vi "Configure Slot.vi"(6 "Delay (sec)":dbl min=0.0 max=99999.999 format="%#.3f", 7 "Number of Poles (1)":enum16{"1", "2", "4"}(ring), 8 "error in":errorcluster, 9 "Card Type (None)":T1(ring), 10 "Slot # (1)":u32=1 min=1 max=2, 11 "VISA resource name":refnum<visa-resource-name>) -> (0 "error out":errorcluster, 3 "VISA resource name out":refnum<visa-resource-name>)   [LabVIEW 2018, in "Keithley 7001.lvlib"]
uses:
  <instrlib>/Keithley 7001/Keithley 7001.lvlib
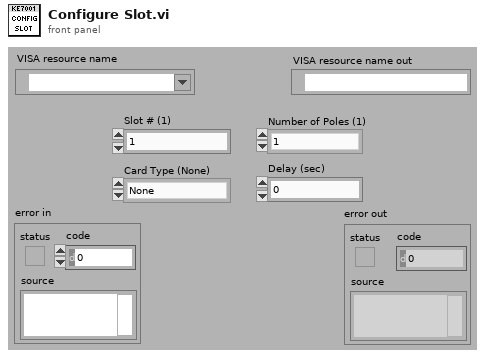
[diagram p1: front panel]
types:
  T1 = enum16{"None", "7052", "7053", "7054", "7056", "7057", "7058", "7059", "7061", "7062", "7063", "7064", "7065", "7066", "7067", "7152", "7153", "7154", "7156", "7158", "7164", "7166", "7168", "7169", "7402", "9990", "9991"}
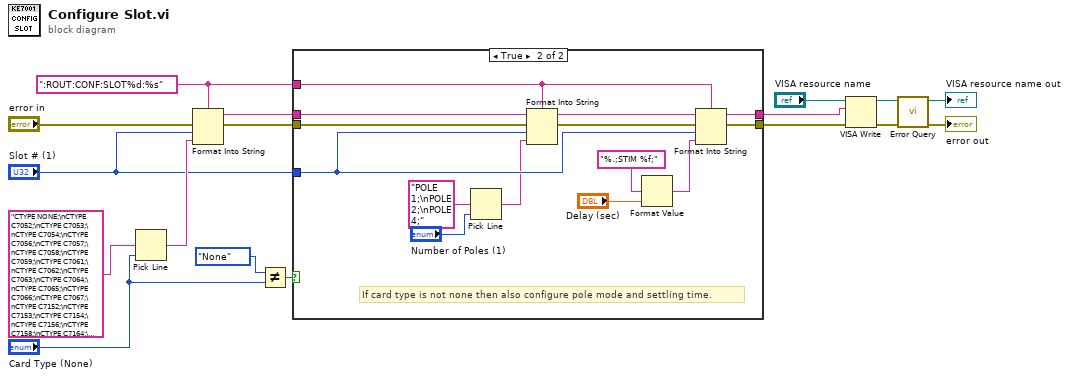
[diagram p0: block diagram]
diagram:
  w8 = ":ROUT:CONF:SLOT%d:%s" ("format string")
  n1 = Pick Line(multi-line string="CTYPE NONE;\nCTYPE C7052;\nCTYPE C7053;\nCTYPE C7054;\nCTYPE C7056;\nCTYPE C7057;\nCTYPE C7058;\nCTYPE C7059;\nCTYPE C7061;\nCTYPE C7062;\nCTYPE C7063;\nCTYPE C7064;\nCTYPE C7065;\nCTYPE C7066;\nCTYPE C7067;\nCTYPE C7152;\nCTYPE C7153;\nCTYPE C7154;\nCTYPE C7156;\nCTYPE C7158;\nCTYPE C7164;\nCTYPE C7166;\nCTYPE C7168;\nCTYPE C7169;\nCTYPE C7402;\nCTYPE C9990;\nCTYPE C9991;", line index="Card Type (None)") -> (output string=w12:string)  [unwired: 1 in]
  n2 = Format Into String(format string=w8, error in="error in", "Slot # (1)", w12) -> (resulting string=w10:string, error out=w9:errorcluster)  [unwired: 1 in]
  n3 = Not Equal?(x=T1."None", y="Card Type (None)") -> (x != y?=w7:bool)
  n4 = case shown="True" w7 {
    tunnel: w10 -> [w19 w30]
    tunnel: w9 -> [w18 w29]
    tunnel: w8 -> [_ w28]
    tunnel: "Slot # (1)" -> [_ w26]
    tunnel: [w19 w22] -> w2
    tunnel: [w18 w20] -> w1
    frame False {
      # "If the card type is None then don't configure pole mode\nor settling time."
    }
    frame True {
      # "If card type is not none then also configure pole mode and settling time."
      n5 = Pick Line(multi-line string="POLE 1;\nPOLE 2;\nPOLE 4;", line index="Number of Poles (1)") -> (output string=w24:string)  [unwired: 1 in]
      n6 = Format Into String(format string=w28, initial string=w30, error in=w29, w26, w24) -> (resulting string=w21:string, error out=w23:errorcluster)
      n7 = Format Value(format string="%.;STIM %f;", value (0)="Delay (sec)") -> (output string=w27:string)  [unwired: 1 in]
      n8 = Format Into String(format string=w28, initial string=w21, error in=w23, w26, w27) -> (resulting string=w22:string, error out=w20:errorcluster)
    }
  }
  n9 = VISA Write(VISA resource name="VISA resource name", write buffer=w2, error in (no error)=w1) -> (VISA resource name out=w15:refnum<visa-resource-name>, error out=w16:errorcluster)  [unwired: 1 out]
  n10 = call <instrlib>:"Error Query.vi"("error in (no error)"=w16, "VISA resource name"=w15) -> ("error out"=→"error out":errorcluster, "VISA resource name out"=→"VISA resource name out":refnum<visa-resource-name>)  [unwired: 6 in, 2 out]
